vi "crio_RT_Load_Cell.vi"() -> ()   [LabVIEW 2019]
uses:
  <vilib>/FPGAPlugInAG/cRIO-9074/niLvFpga_Open_cRIO-9074.vi
  <vilib>/rvi/interface/common/dynamic/niFpgaDynamicAddResources.vi
  <vilib>/Utility/error.llb/Error Cluster From Error Code.vi
  <vilib>/rvi/errors/niLvFpgaAdjustHostInterfaceError.vi
  <vilib>/FPGAPlugInAG/Dynamic/niLvFpga_Close_Dynamic.vi
  <vilib>/rvi/interface/nirviOpenFPGA/nirviOpenFPGA.xnode
  FPGA Bitfiles/gpass2_FPGATarget2_crioFPGALoadCell_XDUAxHyuCEA.lvbitx
  <vilib>/rvi/interface/nirviReadWriteControl/nirviReadWriteControl.xnode
  <vilib>/rvi/interface/nirviCloseFPGA/nirviCloseFPGA.xnode
  NiFpgaLv.dll
  <vilib>/rvi/interface/Simulation/niFpgaSimulationCallBeginRW.vi
panel:
  out "Waveform Chart":dbl(graph)
  out "Mod5/AI0":fxp<+/-,26,5>
  in  "stop":bool
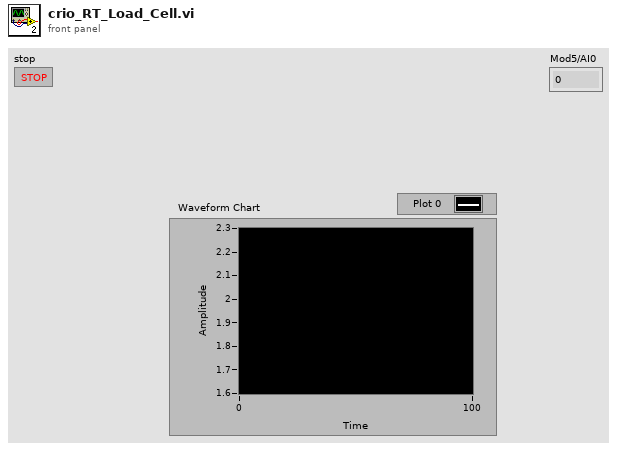
[diagram p1: front panel]
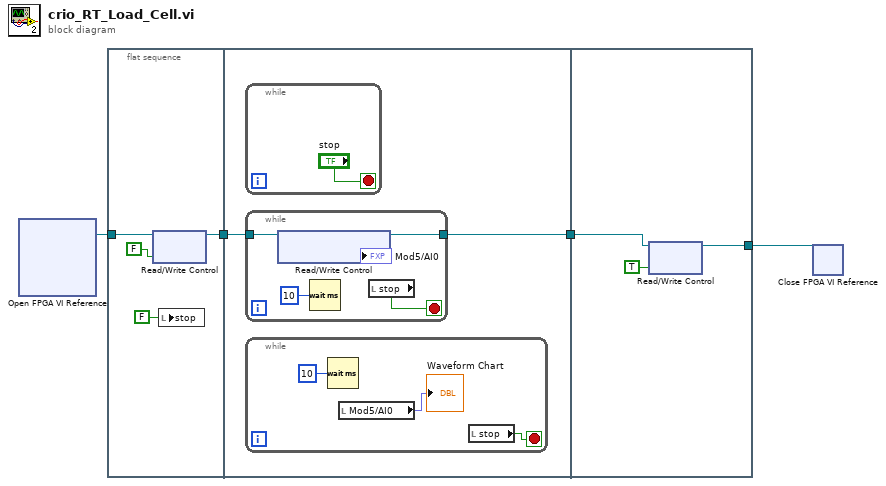
[diagram p0: block diagram]
diagram:
  n1 = xnode "Open FPGA VI Reference"() -> ("FPGA VI Reference Out"=w4:refnum<k20>)  [unwired: 2 in, 1 out]
  n2 = flat-sequence {
    tunnel: w4 -> [w8]
    tunnel: [w6] -> w3
    tunnel: w3 -> [w10]
    tunnel: [w9] -> w2
    tunnel: w2 -> [w22]
    tunnel: [w20] -> w1
    frame #0 {
      n3 = xnode "Read/Write Control"("FPGA VI Reference In"=w8, "stop"=FALSE) -> ("FPGA VI Reference Out"=w6:refnum<k20>)  [unwired: 1 in, 1 out]
      n4 = local write "stop"(FALSE ("stop")) -> ()
    }
    frame #1 {
      n5 = while {
        stop <- "stop" stop-if-true
      }
      n6 = while {
        tunnel: w10 -> [w18]
        tunnel: [w15] -> w9
        stop <- w17 stop-if-true
        n7 = xnode "Read/Write Control"("FPGA VI Reference In"=w18) -> ("FPGA VI Reference Out"=w15:refnum<k20>, "Difference AI2 AI3"=→"Mod5/AI0":fxp<+/-,27,6>)  [unwired: 1 in, 1 out]
        n8 = Wait (ms)(milliseconds to wait=u32 10) -> ()  [unwired: 1 out]
        n9 = local read "stop"() -> (w17:bool)
      }
      n10 = while {
        stop <- w13 stop-if-true
        n11 = Wait (ms)(milliseconds to wait=u32 10) -> ()  [unwired: 1 out]
        n12 = local read "Mod5/AI0"() -> (→"Waveform Chart":fxp<+/-,26,5>)
        n13 = local read "stop"() -> (w13:bool)
      }
    }
    frame #2 {
      n14 = xnode "Read/Write Control"("FPGA VI Reference In"=w22, "stop"=TRUE) -> ("FPGA VI Reference Out"=w20:refnum<k20>)  [unwired: 1 in, 1 out]
    }
  }
  n15 = xnode "Close FPGA VI Reference"("FPGA VI Reference In"=w1) -> ()  [unwired: 1 in, 1 out]
